vi "SVFA Convert Frequency (CPS to CPM).vi"(5 "frequency [Hz]":dbl=100.0) -> (1 "nominal [RPM]":dbl)   [LabVIEW 2017]
doc: "Converts the unit of a rotational speed from revolutions per second, or hertz, to revolutions per minute."
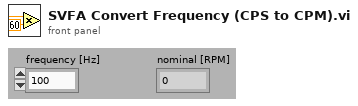
[diagram p1: front panel]
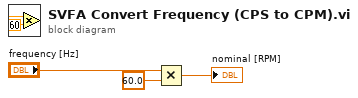
[diagram p0: block diagram]
diagram:
  n1 = Multiply(x="frequency [Hz]", y=60.0) -> (x*y=→"nominal [RPM]":dbl)
